vi "FP - Set Properties_SubVIs-某型振动实验台测试系统.vi"(7 "StateName":string, 8 "error in (no error)":errorcluster, 10 "Controls":refnum<vi>[](array[refnum]), 11 "menu ref":refnum<k9>) -> (0 "error out":errorcluster)   [LabVIEW 2011]
doc: "根据程序所处状态，设置菜单和控件是否可用"
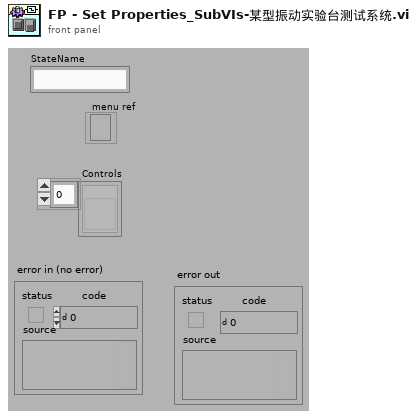
[diagram p1: front panel]
types:
  T1 = enum8{"Enabled", "Disabled", "Disabled and Grayed Out"}
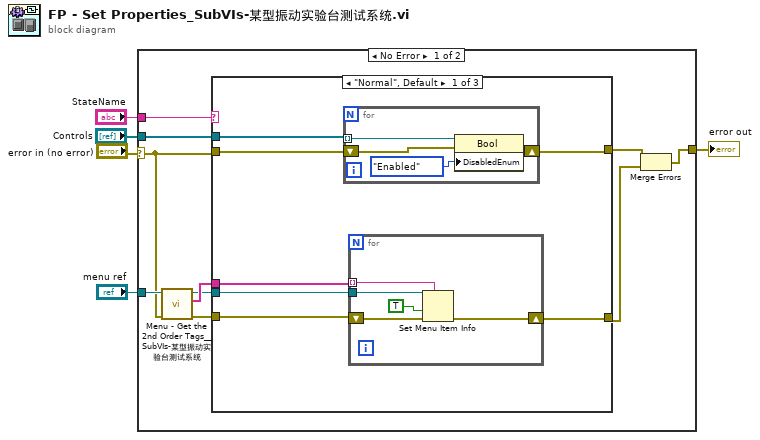
[diagram p0: block diagram]
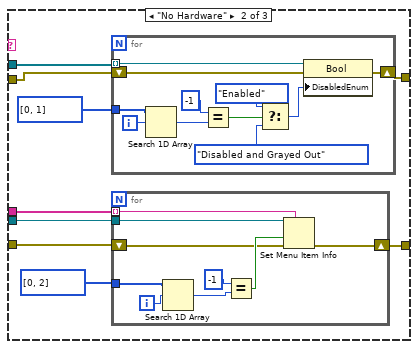
[diagram p2: hidden frame]
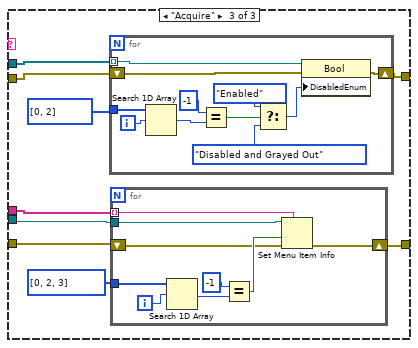
[diagram p3: hidden frame]
diagram:
  n1 = case shown="No Error" "error in (no error)" {
    selector: "error in (no error)" -> [w8 w90]
    tunnel: [w10 w90] -> w2
    tunnel: "StateName" -> [w15 _]
    tunnel: "Controls" -> [w14 _]
    tunnel: "menu ref" -> [w9 _]
    frame No Error {
      n2 = call "Menu - Get the 2nd Order Tags__SubVIs-某型振动实验台测试系统.vi"("error in (no error)"=w8, "menu in"=w9) -> ("error out"=w6:errorcluster, "menu 2nd order tags"=w13:string[], "menu out"=w7:refnum<k9>)  [unwired: 1 in, 6 out]
      n3 = case shown="\"Normal\", Default" w15 {
        tunnel: w14 -> [w22 w40 w68]
        tunnel: w8 -> [w21 w39 w69]
        tunnel: [w20 w38 w67] -> w12
        tunnel: w13 -> [w19 w37 w66]
        tunnel: [w18 w36 w65] -> w11
        tunnel: w7 -> [w17 w33 w62]
        tunnel: w6 -> [w16 w32 w61]
        frame "Normal", Default {
          n4 = for {
            tunnel: w22 -> [w31] mode=indexing
            shift-right: [w28] -> w20
            shift-left: w21 -> [w29]
            n5 = property class="Bool"(reference=w31, error in=w29, "DisabledEnum"=T1."Enabled" ("Disabled")) -> (error out=w28:errorcluster)  [unwired: 1 out]
          }
          n6 = for {
            tunnel: w19 -> [w27] mode=indexing
            shift-right: [w24] -> w18
            shift-left: w16 -> [w25]
            tunnel: w17 -> [w23]
            n7 = Set Menu Item Info(7:w27, 8:w25, 9:TRUE ("enabled"), 11:w23) -> (0:w24:errorcluster)  [unwired: 4 out]
          }
        }
        frame "No Hardware" {
          n8 = for {
            tunnel: w40 -> [w60] mode=indexing
            tunnel: i32[] [0, 1] -> [w52]
            shift-right: [w55] -> w38
            shift-left: w39 -> [w56]
            i -> [w51]
            n9 = Search 1D Array(1D array=w52, element=w51) -> (index of element=w50:i32)  [unwired: 1 out]
            n10 = Equal?(x=-1, y=w50) -> (x = y?=w53:bool)
            n11 = Select(t=T1."Enabled" ("Disabled"), s=w53, f=T1."Disabled and Grayed Out" ("Disabled")) -> (s? t:f=w58:T1)
            n12 = property class="Bool"(reference=w60, error in=w56, "DisabledEnum"=w58) -> (error out=w55:errorcluster)  [unwired: 1 out]
          }
          n13 = for {
            tunnel: i32[] [0, 2] -> [w44]
            tunnel: w37 -> [w47] mode=indexing
            shift-right: [w45] -> w36
            shift-left: w32 -> [w46]
            tunnel: w33 -> [w41]
            i -> [w43]
            n14 = Search 1D Array(1D array=w44, element=w43) -> (index of element=w42:i32)  [unwired: 1 out]
            n15 = Equal?(x=-1, y=w42) -> (x = y?=w48:bool)
            n16 = Set Menu Item Info(7:w47, 8:w46, 9:w48, 11:w41) -> (0:w45:errorcluster)  [unwired: 4 out]
          }
        }
        frame "Acquire" {
          n17 = for {
            tunnel: i32[] [0, 2] -> [w80]
            shift-right: [w85] -> w67
            shift-left: w69 -> [w86]
            tunnel: w68 -> [w81] mode=indexing
            i -> [w79]
            n18 = Search 1D Array(1D array=w80, element=w79) -> (index of element=w83:i32)  [unwired: 1 out]
            n19 = Equal?(x=-1, y=w83) -> (x = y?=w82:bool)
            n20 = Select(t=T1."Enabled" ("Disabled"), s=w82, f=T1."Disabled and Grayed Out" ("Disabled")) -> (s? t:f=w88:T1)
            n21 = property class="Bool"(reference=w81, error in=w86, "DisabledEnum"=w88) -> (error out=w85:errorcluster)  [unwired: 1 out]
          }
          n22 = for {
            tunnel: i32[] [0, 2, 3] -> [w73]
            shift-right: [w75] -> w65
            shift-left: w61 -> [w76]
            tunnel: w66 -> [w74] mode=indexing
            tunnel: w62 -> [w70]
            i -> [w72]
            n23 = Search 1D Array(1D array=w73, element=w72) -> (index of element=w71:i32)  [unwired: 1 out]
            n24 = Equal?(x=-1, y=w71) -> (x = y?=w77:bool)
            n25 = Set Menu Item Info(7:w74, 8:w76, 9:w77, 11:w70) -> (0:w75:errorcluster)  [unwired: 4 out]
          }
        }
      }
      n26 = Merge Errors(w12, w11) -> (w10:errorcluster)
    }
    frame Error {
    }
  }
  "error out" <- w2
